vi "Handle Subpanel VI Run State.vi"(8 "error in (no error)":errorcluster, 11 "VI in":refnum<vi>) -> (0 "error out":errorcluster, 3 "VI out":refnum<vi>)   [LabVIEW 2019, in "Scan Engine Custom Device.lvlib"]
uses:
  Scan Engine Custom Device.lvlib
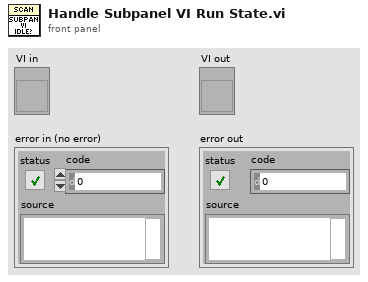
[diagram p1: front panel]
types:
  T1 = enum32{"Bad", "Idle", "Run top level", "Running"}
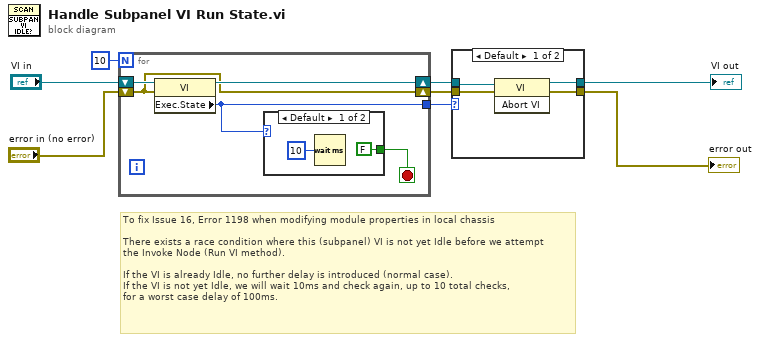
[diagram p0: block diagram]
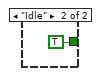
[diagram p3: hidden frame]
diagram:
  # "To fix Issue 16, Error 1198 when modifying module properties in local chassis\n\nThere exists a race condition where this (subpanel) VI is not yet Idle before we attempt\nthe Invoke Node (Run VI method).\n\nIf the VI is already Idle, no further delay is introduced (normal case).\nIf the VI is not yet Idle, we will wait 10ms and check again, up to 10 total checks,\nfor a worst case delay of 100ms."
  n1 = for {
    N: 10 -> [_]
    shift-right: [w11] -> w4
    shift-left: "error in (no error)" -> [w11]
    tunnel: [w10] -> w2
    shift-right: [w12] -> w3
    shift-left: "VI in" -> [w13]
    stop <- w9 stop-if-true
    n2 = property class="VI"(reference=w13, error in=w11) -> (reference out=w12:refnum<vi>, "Exec.State"=w10:T1)  [unwired: 1 out]
    n3 = case shown="Default" w10 {
      tunnel: [FALSE TRUE] -> w9
      frame Default {
        n4 = Wait (ms)(milliseconds to wait=u32 10) -> ()  [unwired: 1 out]
      }
      frame "Idle" {
      }
    }
  }
  n5 = case shown="Default" w2 {
    tunnel: w3 -> [w17 w22]
    tunnel: [w20 w22] -> w8
    tunnel: w4 -> [w18 w21]
    tunnel: [w19 w21] -> w1
    frame Default {
      n6 = invoke class="VI" method="Abort VI"(reference=w17, error in=w18) -> (reference out=w20:refnum<vi>, error out=w19:errorcluster)  [unwired: 1 in, 1 out]
    }
    frame "Idle" {
    }
  }
  "VI out" <- w8
  "error out" <- w1
